vi "AI simulator.vi"(0 "sim I/O info in":T1, 9 "data from node input terminals":variant[](array[variant]), 11 "input from node terminal error in":errorcluster) -> (4 "sim I/O info out":T1, 10 "data to node output terminals":variant[](array[variant]), 15 "output to node terminal error out":errorcluster)   [LabVIEW 2013]
uses:
  <vilib>/FPGA/viExecutionOnDevComputer/simIO/customVI/Sim IO Info.ctl
  <vilib>/rvi/customViForEmulation/niLvFPGAUserSpecifiedEmulationVISupport.lvclass
  <vilib>/FPGA/viExecutionOnDevComputer/simIO/customVI/niFPGA Simulated IO.lvlib
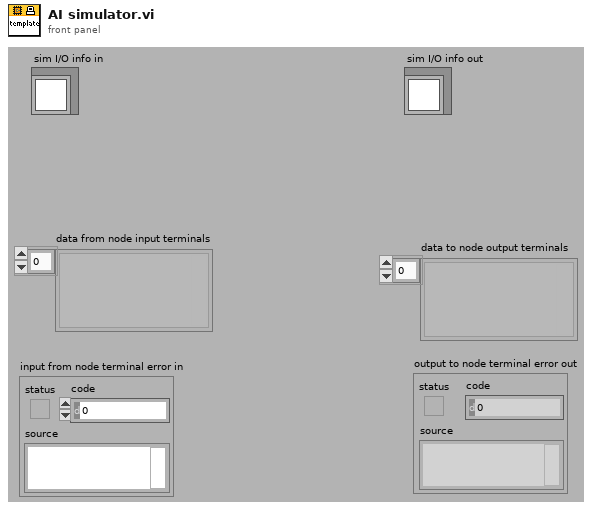
[diagram p1: front panel]
types:
  T1 = typedef "niFPGA Simulated IO.lvlib/Sim IO Info.ctl" = refnum<class "niLvFPGAUserSpecifiedEmulationVISupport.lvclass">
  T2 = typedef "niFPGA Simulated IO.lvlib/Execution Stage.ctl" = enum16{"Initializing", "Running", "Shutting Down"}
  T3 = typedef "niFPGA Simulated IO.lvlib/Node or Element Type.ctl" = enum16{"Read I/O", "Write I/O", "Method", "Read Property", "Write Property"}
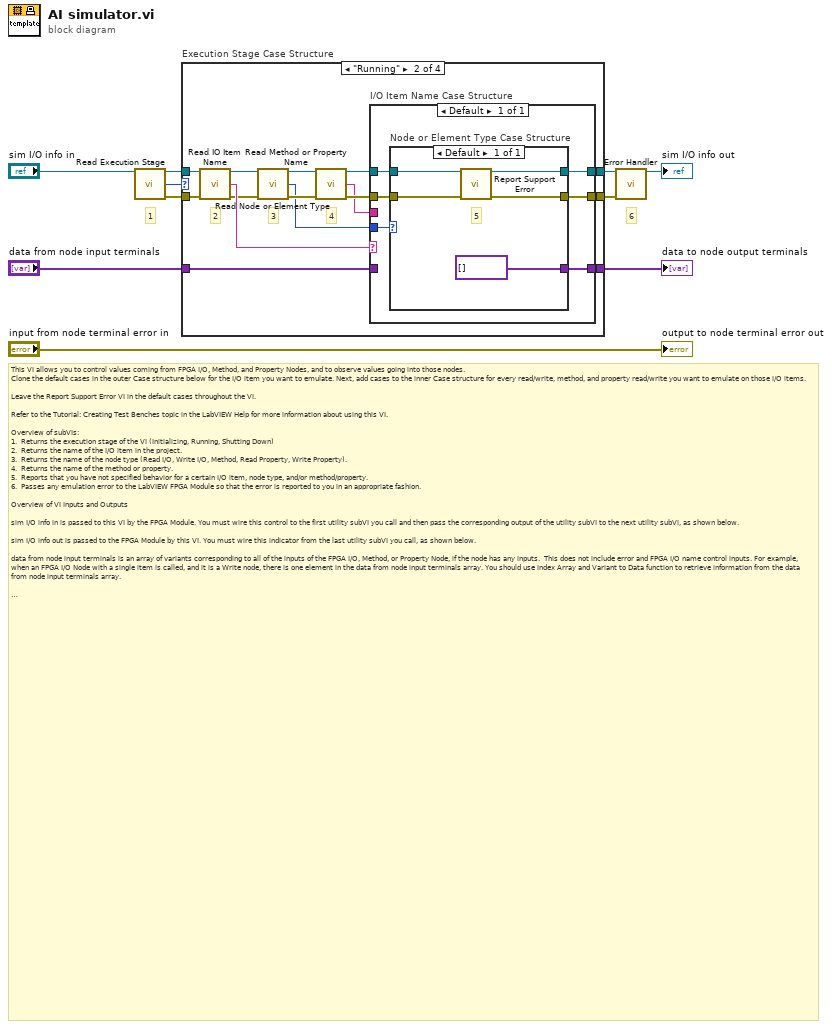
[diagram p0: block diagram]
diagram:
  # "1"
  # "6"
  # "This VI allows you to control values coming from FPGA I/O, Method, and Property Nodes, and to observe values going into those nodes.\nClone the default cases in the outer Case structure below for the I/O item you want to emulate. Next, add cases to the inner Case structure for every read/write, method, and property read/write you want to emulate on those I/O items.  \n\nLeave the Report Support Error VI in the default cases throughout the VI.\n\nRefer to the Tutorial: Creating Test Benches topic in the LabVIEW Help for more information about using this VI.\n\nOverview of subVIs:\n1.  Returns the execution stage of the VI (Initializing, Running, Shutting Down)\n2.  Returns the name of the I/O item in the project.\n3.  Returns the name of the node type (Read I/O, Write I/O, Method, Read Property, Write Property).\n4.  Returns the name of the method or property.\n5.  Reports that you have not specified behavior for a certain I/O item, node type, and/or method/property.\n6.  Passes any emulation error to the LabVIEW FPGA Module so that the error is reported to you in an appropriate fashion.\n\nOverview of VI Inputs and Outputs\n\nsim I/O info in is passed to this VI by the FPGA Module. You must wire this control to the first utility subVI you call and then pass the corresponding output of the utility subVI to the next utility subVI, as shown below.\n\nsim I/O info out is passed to the FPGA Module by this VI. You must wire this indicator from the last utility subVI you call, as shown below.\n\ndata from node input terminals is an array of variants corresponding to all of the inputs of the FPGA I/O, Method, or Property Node, if the node has any inputs.  This does not include error and FPGA I/O name control inputs. For example, when an FPGA I/O Node with a single item is called, and it is a Write node, there is one element in the data from node input terminals array. You should use Index Array and Variant to Data function to retrieve information from the data from node input terminals array.\n\ndata to node output terminals is an array of variants corresponding to all the outputs of the FPGA I/O, Method, or Property Node, if the node has any outputs.  This does not include error and FPGA I/O name control outputs. For example, when an FPGA I/O node with a single item is called, and it is a Read node, there should be one element in the data to node output terminals array. You should use To Variant and Build Array functions to pass the information to the data to node output terminals array.\n\ninput from node terminal error in is the error that gets passed into the FPGA I/O, Method, or Property Node, if the node is configured so that the error input is shown. If the node is configured so that the error input is not shown, the value of this input corresponds to \"no error\" (status is false, error code is 0). \n\noutput to node terminal error out is the error that gets passed out of the FPGA I/O, Method, or Property Node, if the node is configured so that the error output is shown.  If the node is configured so that the error output is not shown, the value of this output is ignored."
  n1 = call <vilib>:"Read Execution Stage.vi"("sim I/O info in"="sim I/O info in") -> ("sim I/O info out"=w3:T1, "execution stage"=w1:T2, "error out"=w2:errorcluster)  [unwired: 1 in, 11 out]
  n2 = case "Execution Stage Case Structure" shown="\"Running\"" w1 {
    tunnel: [_ w26 _ _] -> w9
    tunnel: [w12 w21 w40 w42] -> w4
    tunnel: [w11 w17 w39 w41] -> w6
    tunnel: w3 -> [w11 w15 w39 w41]
    tunnel: w2 -> [w12 w14 w40 w42]
    tunnel: "data from node input terminals" -> [_ w27 _ _]
    frame "Initializing" {
    }
    frame "Running" {
      # "4"
      # "3"
      # "2"
      n3 = call <vilib>:"Read IO Item Name.vi"("sim I/O info in"=w15, "error in (no error)"=w14) -> ("sim I/O info out"=w16:T1, "I/O item name"=w25:string, "error out"=w24:errorcluster)  [unwired: 11 out]
      n4 = call <vilib>:"Read Node or Element Type.vi"("sim I/O info in"=w16, "error in (no error)"=w24) -> ("sim I/O info out"=w13:T1, "node or element type"=w22:T3, "error out"=w23:errorcluster)  [unwired: 11 out]
      n5 = call <vilib>:"Read Method or Property Name.vi"("sim I/O info in"=w13, "error in (no error)"=w23) -> ("sim I/O info out"=w19:T1, "method or property name"=w18:string, "error out"=w20:errorcluster)  [unwired: 11 out]
      n6 = case "I/O Item Name Case Structure" shown="Default" w25 {
        tunnel: w27 -> [_]
        tunnel: [w29] -> w26
        tunnel: w20 -> [w33]
        tunnel: [w32] -> w21
        tunnel: w19 -> [w31]
        tunnel: [w30] -> w17
        tunnel: w22 -> [w28]
        tunnel: w18 -> [_]
        frame Default {
          n7 = case "Node or Element Type Case Structure" shown="Default" w28 {
            tunnel: w33 -> [w38]
            tunnel: [w37] -> w32
            tunnel: w31 -> [w36]
            tunnel: [w35] -> w30
            tunnel: [variant[] []] -> w29
            frame Default {
              # "5"
              n8 = call <vilib>:"Report Support Error.vi"("sim I/O info in"=w36, "error in (no error)"=w38) -> ("sim I/O info out"=w35:T1, "error out"=w37:errorcluster)  [unwired: 12 out]
            }
          }
        }
      }
    }
    frame "Shutting Down" {
    }
    frame Default {
    }
  }
  "data to node output terminals" <- w9
  n9 = call <vilib>:"Error Handler.vi"("sim I/O info in"=w6, "error in"=w4) -> ("sim I/O info out"=→"sim I/O info out":T1)  [unwired: 13 out]
  "output to node terminal error out" <- "input from node terminal error in"
